vi "Check if configuration files exist.vi"(8 "error in (no error)":errorcluster, 11 "ExampleClassB in":refnum<class "ExampleClassB.lvclass">) -> (0 "error out":errorcluster, 2 "configuration file exists?":bool, 3 "ExampleClassB out":refnum<class "ExampleClassB.lvclass">)   [LabVIEW 2012, in "ExampleClassB.lvclass"]
doc: "Checks whether all required configuration files for the component exist."
uses:
  ExampleClassB.lvclass
  <vilib>/Distrio/Murmex/Murmex/Murmex.lvclass
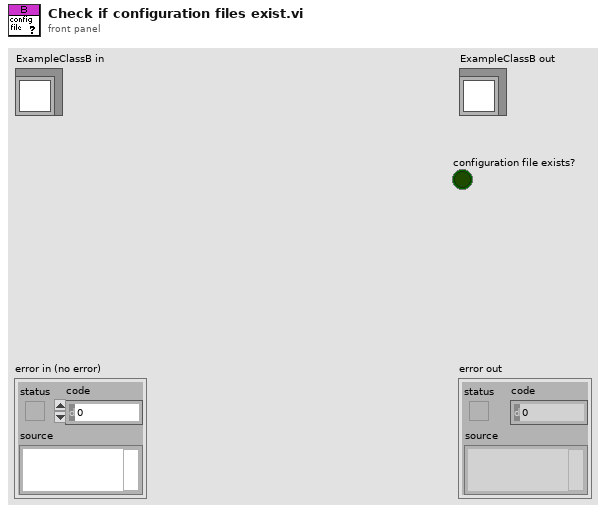
[diagram p1: front panel]
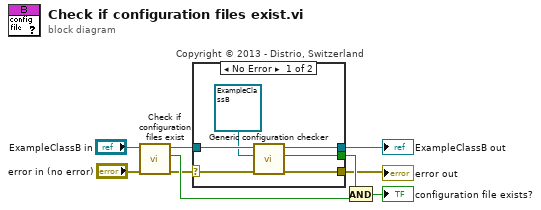
[diagram p0: block diagram]
diagram:
  n1 = call-parent "Check if configuration files exist.vi"("error in (no error)"="error in (no error)", "Murmex in"="ExampleClassB in") -> ("error out"=w5:errorcluster, "configuration file exists?"=w7:bool, "Murmex out"=w4:refnum<class "ExampleClassB.lvclass">)  [unwired: 7 in]
  n2 = case "Copyright © 2013 - Distrio, Switzerland" shown="No Error" w5 {
    selector: w5 -> [w15 w17]
    tunnel: [w13 w17] -> w1
    tunnel: [w11 w16] -> w3
    tunnel: w4 -> [w14 w16]
    tunnel: [w12 _] -> w2
    frame No Error {
      n3 = call <vilib>:"Generic configuration checker.vi"("error in (no error)"=w15, "inheritance level"=refnum<class "ExampleClassB.lvclass"> refnum ("ExampleClassB"), "Murmex in"=w14) -> ("error out"=w13:errorcluster, "configuration file exists?"=w12:bool, "Murmex out"=w11:refnum<class "ExampleClassB.lvclass">)  [unwired: 6 in]
    }
    frame Error {
    }
  }
  "error out" <- w1
  "ExampleClassB out" <- w3
  n4 = And(x=w2, y=w7) -> (x .and. y?=→"configuration file exists?":bool)
